vi "SwitchToAnalogOrDigital.vi"(0 "System no.":i32=1 min=1 step=1, 1 "Controller analog board":enum16{"E-711.iA4"}(ring), 2 "Axes to command":string[](array[string]), 3 "Mode":bool=TRUE caption="Mode (Analog:T)", 5 "error in":errorcluster, 6 "AI channels":dbl[](array[numeric]), 7 "AO channels":dbl[](array[numeric]), 8 "Lower voltage limit (V)":dbl=-10.0 format="%.6f", 9 "Upper voltage limit (V)":dbl=10.0 format="%.6f") -> (14 "Conversion factor":dbl[](array[numeric]) format="%.2f", 15 "Offset":dbl[](array[numeric]) format="%#.6f", 19 "Error out":errorcluster)   [LabVIEW 2026]
doc: "This VI sets communication parameters for analog or digital control. Run PI_GCS2_Configuration_Setup.vi prior to running this VI. \n\n- Set System no. to the same value as selected in PI_GCS2_Configuration_Setup.vi. \n- Select the name of the controller analog board (E-711.iA4).\n- Mode can be Analog (T) or Digital (F). \n- Lower voltage limit (V) and Upper voltage limit (V) must match the corresponding settings in Analog_Configuration_Setup.vi, representing the voltage range of the analog input of the controller. The VI checks if the selected values fit into the analog input voltage range of the controller. \n- Axes to command must be a sub set of the axes connected to the controller. \n- AI channels are the analog input channels of the controller to use for analog control. In contrast to the firmware internal names of the analog input channels, select \"1\" here for the first analog input, \"2\" for the second and so on. The VI will automatically determine which input channel names correspond to the selected analog input channels. \n- Similarly, select \"1\" for the first analog output channel (AO channels), \"2\" for the second analog output channel and so on, as the VI will automatically determine which output channel names correspond to the selected analog output channels. \n\nIf the current command level is 0 (CCL?), the VI switches to command level 1 (CCL) before making any further settings and back to 0 afterwards. \nWhen Analog is selected as Mode, the VI connects the selected analog input channels to the selected axes (SPA), sets gain and offset for the analog input (SPA), sets the output type to sensor monitor output (SPA), connects the selected analog output channels to the selected axes (SPA), and sets the position report scaling value and offset for the analog output (SPA).\nWhen Digital is selected as Mode, the VI disconnects the selected analog input channels from the axes (SPA) and sets the output type to control output (SPA).\nThe VI returns the total number of input and output channels available for this controller, the number of sensor input/output channels and the resulting number of analog input/output channels available for analog control. Also, it returns the Gain, Offset and Conversion factor settings resulting from the motion range (TMX?, TMN?) of the selected axes and sets the corresponding parameters (SPA). Finally, it returns the minimum and maximum analog input voltages of the controller as the given lower and upper voltage limits must fit into this range.\n\nSee XXXX_Sample_Application_With_Analog.vi as a sample VI showing how to use this VI in combination with the corresponding Configuration_Setup VIs."
panel:
  out "Max. controller\nanalog input voltage":dbl format="%#.6f"
  out "Min. controller\nanalog input voltage":dbl format="%#.6f"
  out "Gain":dbl[](array[numeric]) format="%#.6f"
  out "No. of output channels":dbl format="%#.0f"
  out "No. of sensor output channels":dbl format="%#.0f"
  out "No. of AO channels":dbl format="%#.0f"
  out "No. of AI channels":dbl format="%#.0f"
  out "No. of sensor input channels":dbl format="%#.0f"
  out "No. of input channels":dbl format="%#.0f"
  # "This VI sets communication parameters for analog or digital control. Run XXXX_Configuration_Setup.vi (with XXXX being the product number of your PI controller) prior to running this VI. Set System no. to the same value as selected in XXXX_Configuration_Setup.vi. See online help for details."
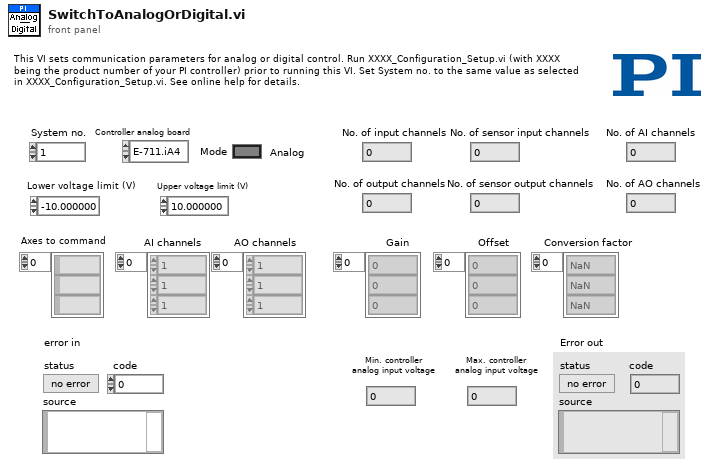
[diagram p1: front panel]
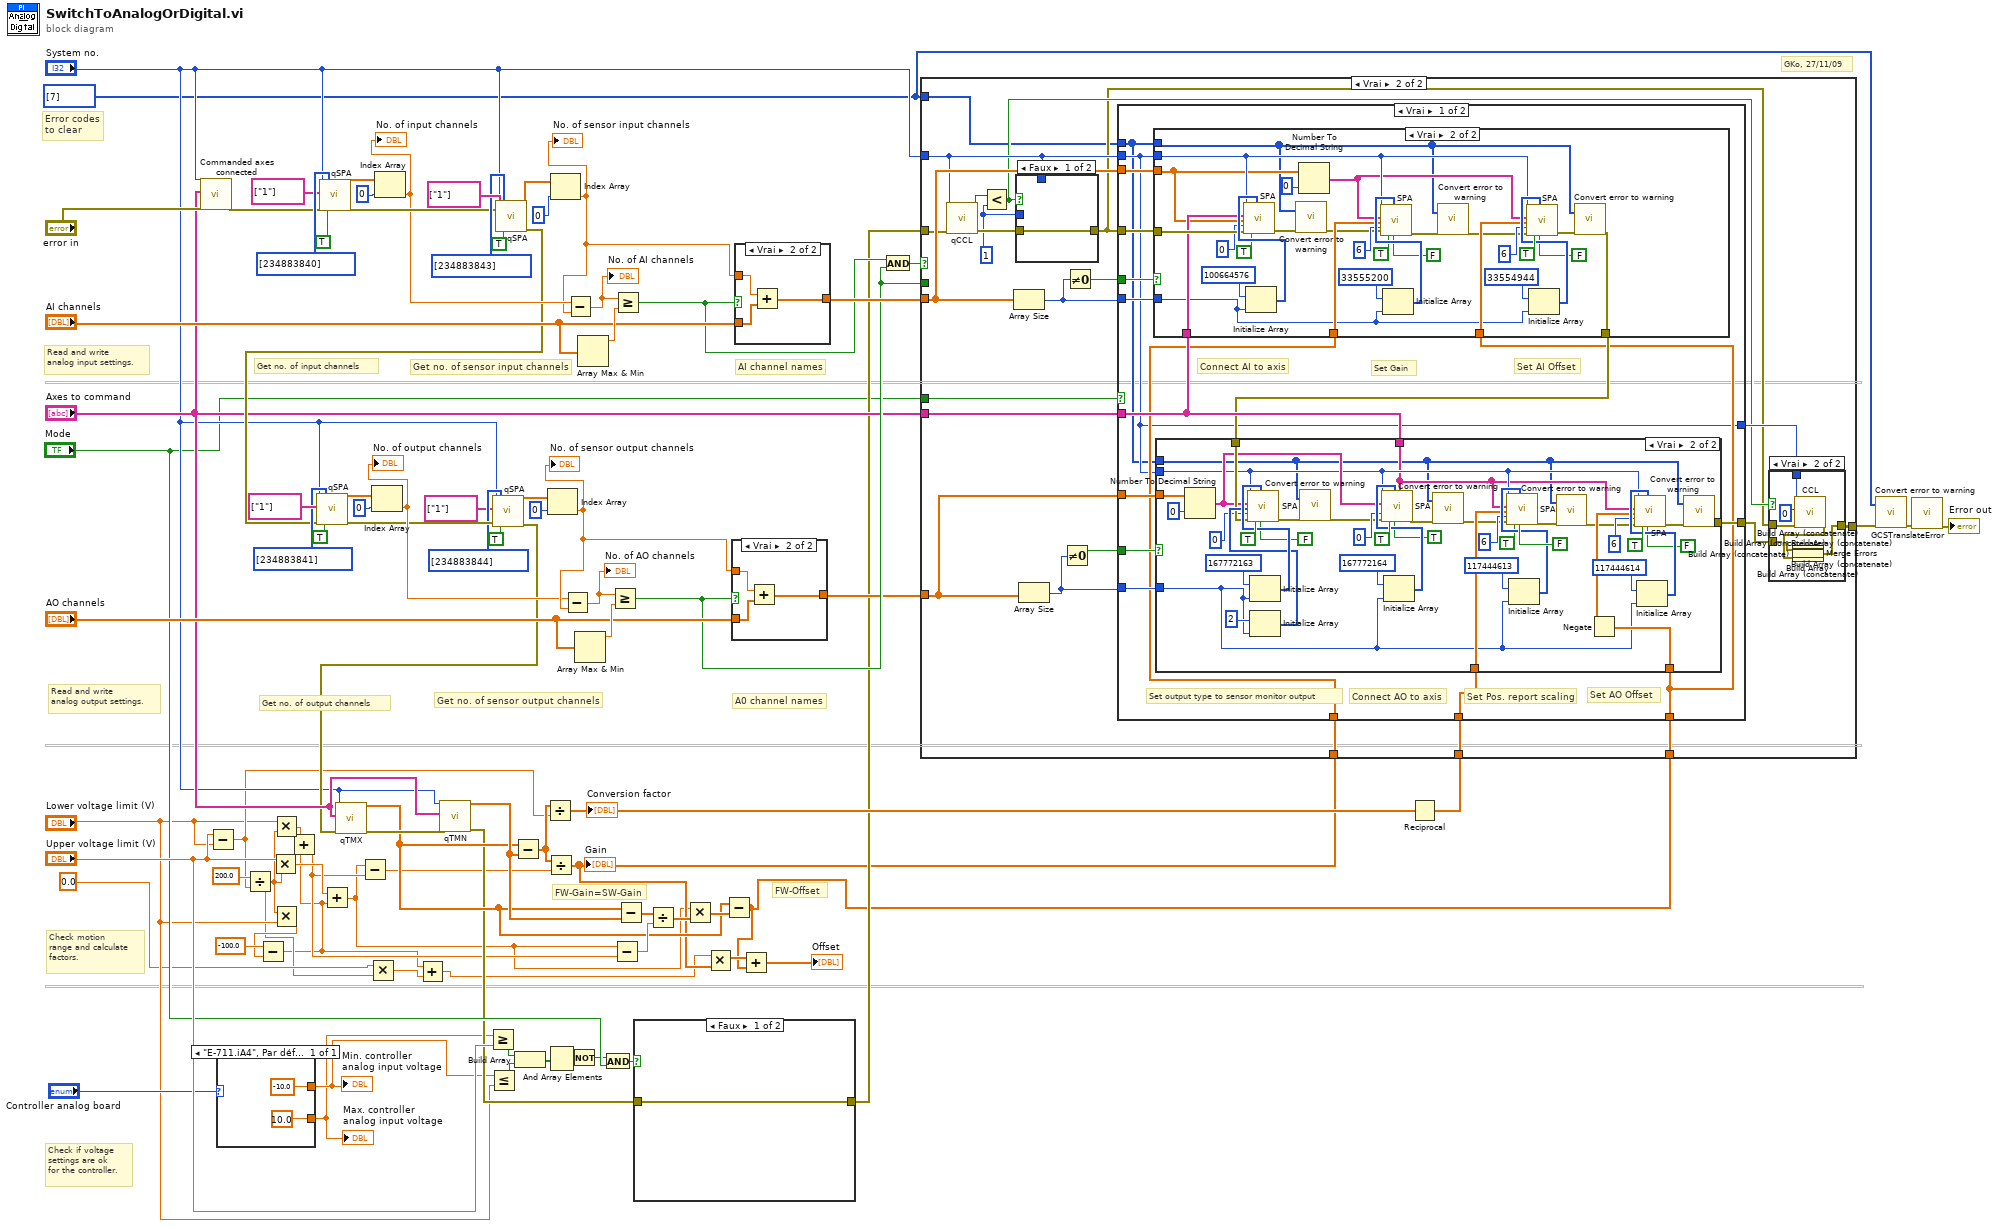
[diagram p0: block diagram]
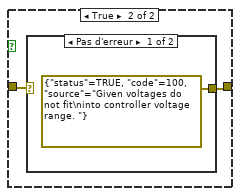
[diagram p2: hidden frame]
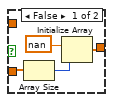
[diagram p4: hidden frame]
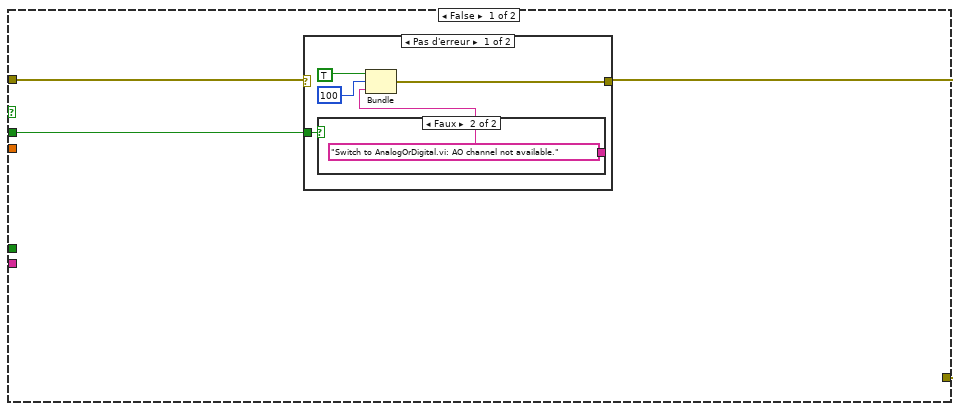
[diagram p5: hidden frame]
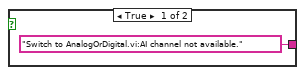
[diagram p6: hidden frame]
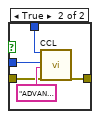
[diagram p9: hidden frame]
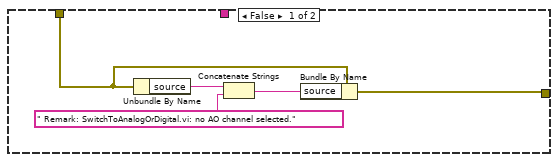
[diagram p10: hidden frame]
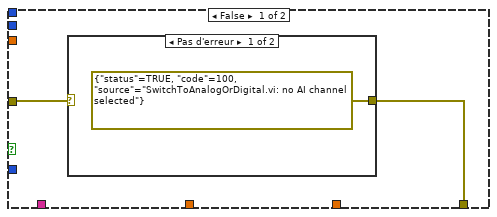
[diagram p11: hidden frame]
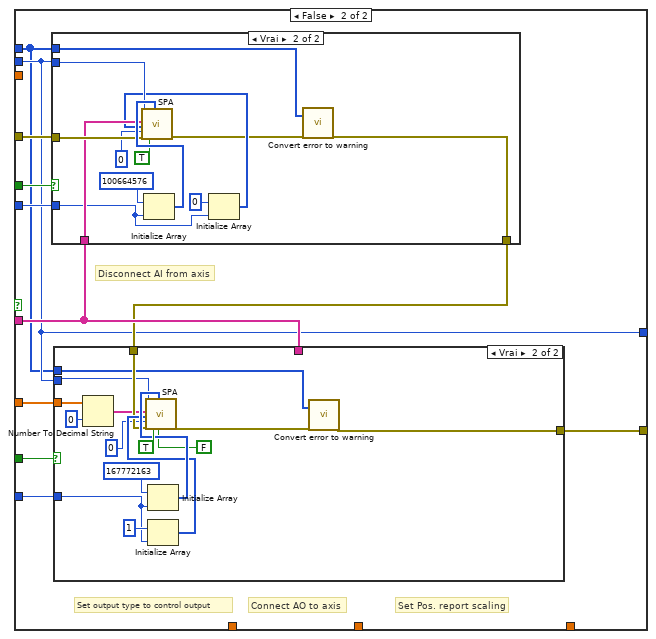
[diagram p13: hidden frame]
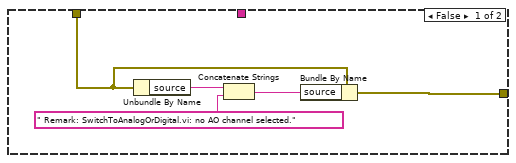
[diagram p14: hidden frame]
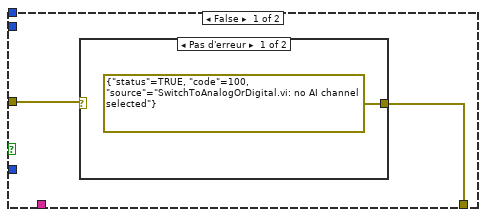
[diagram p15: hidden frame]
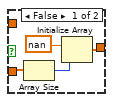
[diagram p17: hidden frame]
diagram:
  w20 = i32[] [7] ("Codes")
  # "Error codes\nto clear"
  # "Get no. of sensor output channels"
  # "Get no. of output channels"
  # "Get no. of sensor input channels"
  # "Get no. of input channels"
  # "FW-Offset"
  # "FW-Gain=SW-Gain"
  # "A0 channel names"
  # "GKo, 27/11/09"
  # "Read and write\nanalog output settings."
  # "Check motion\nrange and calculate\nfactors."
  # "Check if voltage\nsettings are ok\nfor the controller."
  # "AI channel names"
  # "Read and write\nanalog input settings."
  n1 = call "Commanded axes connected.vi"("System no."="System no.", "Commanded axes"="Axes to command", "error in"="error in") -> ("error out"=w73:errorcluster)  [unwired: 16 out]
  n2 = Subtract(x="Upper voltage limit (V)", y="Lower voltage limit (V)") -> (x-y=w18:dbl)
  n3 = case shown="\"E-711.iA4\", Par défaut" "Controller analog board" {
    tunnel: [-10.0 ("y")] -> w25
    tunnel: [10.0 ("y")] -> w24
    frame "E-711.iA4", Default {
    }
  }
  "Min. controller\nanalog input voltage" <- w25
  "Max. controller\nanalog input voltage" <- w24
  n4 = Divide(x=200.0, y=w18) -> (x/y=w3:dbl)
  n5 = Multiply(x="Upper voltage limit (V)", y=w3) -> (x*y=w13:dbl)
  n6 = Multiply(x="Lower voltage limit (V)", y=w3) -> (x*y=w14:dbl)
  n7 = Multiply(x=w3, y="Lower voltage limit (V)") -> (x*y=w15:dbl)
  n8 = Subtract(x=-100.0, y=w15) -> (x-y=w2:dbl)
  n9 = Add(x=w14, y=w2) -> (x+y=w7:dbl)
  n10 = call "qSPA.vi"("System no."="System no.", "Axes to query"=string[] ["1"], "error in"=w73, "Parameter no. (hex)"=u32[] [234883840], "Parameter no. format \n(Decimal: FALSE)"=TRUE ("Parameter no. format \n(Decimal: FALSE)")) -> ("Parameter value"=w86:dbl[], "error out"=w79:errorcluster)  [unwired: 2 in, 11 out]
  n11 = Add(x=w13, y=w2) -> (x+y=w6:dbl)
  n12 = Subtract(x=w6, y=w7) -> (x-y=w4:dbl)
  n13 = Multiply(x=0.0, y=w3) -> (x*y=w5:dbl)
  n14 = Index Array(array=w86, index=0) -> (element=w78:dbl)
  "No. of input channels" <- w78
  n15 = Add(x=w2, y=w5) -> (x+y=w1:dbl)
  n16 = Greater Or Equal?(x=w24, y="Upper voltage limit (V)") -> (x >= y?=w35:bool)
  n17 = Less Or Equal?(x=w25, y="Lower voltage limit (V)") -> (x <= y?=w34:bool)
  n18 = call "qSPA.vi"("System no."="System no.", "Axes to query"=string[] ["1"], "error in"=w79, "Parameter no. (hex)"=u32[] [234883843], "Parameter no. format \n(Decimal: FALSE)"=TRUE ("Parameter no. format \n(Decimal: FALSE)")) -> ("Parameter value"=w83:dbl[], "error out"=w55:errorcluster)  [unwired: 2 in, 11 out]
  n19 = call "qSPA.vi"("System no."="System no.", "Axes to query"=string[] ["1"], "error in"=w55, "Parameter no. (hex)"=u32[] [234883841], "Parameter no. format \n(Decimal: FALSE)"=TRUE ("Parameter no. format \n(Decimal: FALSE)")) -> ("Parameter value"=w59:dbl[], "error out"=w66:errorcluster)  [unwired: 2 in, 11 out]
  n20 = Index Array(array=w59, index=0) -> (element=w67:dbl)
  "No. of output channels" <- w67
  n21 = call "qSPA.vi"("System no."="System no.", "Axes to query"=string[] ["1"], "error in"=w66, "Parameter no. (hex)"=u32[] [234883844], "Parameter no. format \n(Decimal: FALSE)"=TRUE ("Parameter no. format \n(Decimal: FALSE)")) -> ("Parameter value"=w62:dbl[], "error out"=w49:errorcluster)  [unwired: 2 in, 11 out]
  n22 = call "qTMX.vi"("System no."="System no.", "Axes to query"="Axes to command", "error in"=w49) -> ("Maximum travel limit"=w42:dbl[], "error out"=w48:errorcluster)  [unwired: 2 in, 13 out]
  n23 = call "qTMN.vi"("System no."="System no.", "Axes to query"="Axes to command", "error in"=w48) -> ("Minimum travel limit"=w47:dbl[], "error out"=w26:errorcluster)  [unwired: 2 in, 13 out]
  n24 = Subtract(x=w42, y=w47) -> (x-y=w41:dbl[])
  n25 = Build Array(w35, w34) -> (w33:bool[])
  n26 = Divide(x=w41, y=w18) -> (x/y=w40:dbl[])
  "Conversion factor" <- w40
  n27 = Divide(x=w41, y=w4) -> (x/y=w12:dbl[])
  "Gain" <- w12
  n28 = And Array Elements(Boolean array=w33) -> (logical AND=w30:bool)
  n29 = Index Array(array=w62, index=0) -> (element=w68:dbl)
  "No. of sensor output channels" <- w68
  n30 = Index Array(array=w83, index=0) -> (element=w77:dbl)
  "No. of sensor input channels" <- w77
  n31 = Subtract(x=w67, y=w68) -> (x-y=w69:dbl)
  "No. of AO channels" <- w69
  n32 = Subtract(x=w78, y=w77) -> (x-y=w76:dbl)
  "No. of AI channels" <- w76
  n33 = Not(x=w30) -> (.not. x?=w28:bool)
  n34 = Array Max & Min(array="AO channels") -> (max value=w70:dbl)  [unwired: 3 out]
  n35 = Array Max & Min(array="AI channels") -> (max value=w75:dbl)  [unwired: 3 out]
  n36 = And(x=w28, y="Mode") -> (x .and. y?=w27:bool)
  n37 = Greater Or Equal?(x=w69, y=w70) -> (x >= y?=w51:bool)
  n38 = Subtract(x=w6, y=w7) -> (x-y=w45:dbl)
  n39 = Greater Or Equal?(x=w76, y=w75) -> (x >= y?=w53:bool)
  n40 = Subtract(x=w42, y=w47) -> (x-y=w46:dbl[])
  n41 = case shown="Faux" w27 {
    tunnel: w26 -> [w92 w94]
    tunnel: [w92 w93] -> w32
    frame False {
    }
    frame True {
      n42 = case shown="Pas d'erreur" w94 {
        selector: w94 -> [_ w96]
        tunnel: [errorcluster {"status"=TRUE, "code"=100, "source"="Given voltages do not fit\ninto controller voltage range. "} ("error IO") w96] -> w93
        frame No Error {
        }
        frame Error {
        }
      }
    }
  }
  n43 = Divide(x=w46, y=w45) -> (x/y=w44:dbl[])
  n44 = Multiply(x=w6, y=w44) -> (x*y=w43:dbl[])
  n45 = Multiply(x=w1, y=w12) -> (x*y=w11:dbl[])
  n46 = Subtract(x=w42, y=w43) -> (x-y=w10:dbl[])
  n47 = case shown="Vrai" w51 {
    tunnel: "AO channels" -> [w100 w102]
    tunnel: w68 -> [_ w103]
    tunnel: [w97 w101] -> w38
    frame False {
      n48 = Array Size(array=w100) -> (size(s)=w98:i32)
      n49 = Initialize Array(nan, w98) -> (w97:dbl[])
    }
    frame True {
      n50 = Add(x=w103, y=w102) -> (x+y=w101:dbl[])
    }
  }
  n51 = case shown="Vrai" w53 {
    tunnel: "AI channels" -> [w107 w109]
    tunnel: w77 -> [_ w110]
    tunnel: [w104 w108] -> w71
    frame False {
      n52 = Array Size(array=w107) -> (size(s)=w105:i32)
      n53 = Initialize Array(nan, w105) -> (w104:dbl[])
    }
    frame True {
      n54 = Add(x=w110, y=w109) -> (x+y=w108:dbl[])
    }
  }
  n55 = Add(x=w11, y=w10) -> (x+y=→"Offset":dbl[])
  n56 = And(x=w53, y=w51) -> (x .and. y?=w52:bool)
  n57 = Reciprocal(x=w40) -> (1/x=w39:dbl[])
  n58 = case shown="Vrai" w52 {
    tunnel: "System no." -> [_ w128]
    tunnel: w71 -> [_ w133]
    tunnel: "Axes to command" -> [_ w142]
    tunnel: w32 -> [w113 w129]
    tunnel: w51 -> [w112 _]
    tunnel: w38 -> [_ w143]
    tunnel: w12 -> [_ w136]
    tunnel: w10 -> [_ w135]
    tunnel: [w111 w132] -> w22
    tunnel: w39 -> [_ w141]
    tunnel: "Mode" -> [_ w134]
    tunnel: w20 -> [_ w122]
    frame False {
      n59 = case shown="Pas d'erreur" w113 {
        selector: w113 -> [_ w121]
        tunnel: w112 -> [w116 _]
        tunnel: [w114 w121] -> w111
        frame No Error {
          n60 = case shown="Faux" w116 {
            tunnel: ["Switch to AnalogOrDigital.vi:AI channel not available." ("source") "Switch to AnalogOrDigital.vi: AO channel not available." ("source")] -> w115
            frame True {
            }
            frame False {
            }
          }
          n61 = Bundle("status"=TRUE, "code"=100, "source"=w115) -> (w114:errorcluster)  [unwired: 1 out]
        }
        frame Error {
        }
      }
    }
    frame True {
      w126 = 1 ("Command level")
      n62 = call "qCCL.vi"("System no."=w128, "error in"=w129) -> ("Command level"=w127:i32, "error out"=w130:errorcluster)  [unwired: 16 out]
      n63 = Less?(x=w127, y=w126) -> (x < y?=w125:bool)
      n64 = Array Size(array=w133) -> (size(s)=w139:i32)
      n65 = case shown="Faux" w125 {
        tunnel: [w158 w163] -> w124
        tunnel: w130 -> [w158 w161]
        tunnel: w128 -> [_ w160]
        tunnel: w126 -> [_ w159]
        frame False {
        }
        frame True {
          n66 = call "CCL.vi"("System no."=w160, "Command level"=w159, "Password"="ADVANCED", "error in"=w161) -> ("error out"=w163:errorcluster)  [unwired: 15 out]
        }
      }
      n67 = Array Size(array=w143) -> (size(s)=w138:i32)
      n68 = Not Equal To 0?(x=w138) -> (x != 0?=w137:bool)
      n69 = Not Equal To 0?(x=w139) -> (x != 0?=w140:bool)
      n70 = case shown="Vrai" w134 {
        tunnel: w124 -> [w178 w269]
        tunnel: w143 -> [w177 w268]
        tunnel: [w176 w267] -> w123
        tunnel: w142 -> [w175 w266]
        tunnel: w141 -> [w174 _]
        tunnel: w128 -> [w165 w260]
        tunnel: w133 -> [w172 _]
        tunnel: w140 -> [w171 w264]
        tunnel: w139 -> [w170 w263]
        tunnel: w138 -> [w169 w262]
        tunnel: w137 -> [w168 w261]
        tunnel: w136 -> [w167 _]
        tunnel: w135 -> [w166 _]
        tunnel: [w165 w260] -> w131
        tunnel: w122 -> [w164 w259]
        frame True {
          # "Set AO Offset"
          # "Set Pos. report scaling"
          # "Set AI Offset"
          # "Set Gain"
          # "Connect AO to axis"
          # "Set output type to sensor monitor output"
          # "Connect AI to axis"
          n71 = case shown="Vrai" w171 {
            tunnel: w178 -> [w226 w256]
            tunnel: w167 -> [_ w251]
            tunnel: w166 -> [_ w245]
            tunnel: w175 -> [_ w244]
            tunnel: [w225 w230] -> w173
            tunnel: w165 -> [_ w243]
            tunnel: w170 -> [_ w242]
            tunnel: w172 -> [_ w240]
            tunnel: w164 -> [_ w229]
            frame False {
              n72 = case shown="Pas d'erreur" w226 {
                selector: w226 -> [_ w228]
                tunnel: [errorcluster {"status"=TRUE, "code"=100, "source"="SwitchToAnalogOrDigital.vi: no AI channel selected"} ("error IO") w228] -> w225
                frame No Error {
                }
                frame Error {
                }
              }
            }
            frame True {
              n73 = Initialize Array(100664576 ("Numeric"), w242) -> (w257:i32[])
              n74 = call "SPA.vi"("System no."=w243, "Axis to set"=w244, "Parameter value"=w240, "No.of digits"=i16 0, "error in"=w256, "Parameter no. format \n(Decimal: FALSE)"=TRUE ("Parameter no. format \n(Decimal: FALSE)"), "Parameter number (hex)"=w257) -> ("error out"=w235:errorcluster)  [unwired: 3 in, 9 out]
              n75 = call "Convert error to warning.vi"("Codes"=w229, "error in"=w235) -> ("error out"=w234:errorcluster)  [unwired: 17 out]
              n76 = Number To Decimal String(number=w240, width (-)=i16 0) -> (decimal integer string=w241:string[])
              n77 = Initialize Array(33555200 ("Numeric"), w242) -> (w253:i32[])
              n78 = call "SPA.vi"("System no."=w243, "Axis to set"=w241, "Parameter value"=w251, "No.of digits"=i16 6, "error in"=w234, "Parameter no. format \n(Decimal: FALSE)"=TRUE ("Parameter no. format \n(Decimal: FALSE)"), "Parameter number (hex)"=w253, "Parameter format \n(Num.: FALSE)"=FALSE ("Parameter format \n(Num.: FALSE)")) -> ("error out"=w233:errorcluster)  [unwired: 2 in, 9 out]
              n79 = call "Convert error to warning.vi"("Codes"=w229, "error in"=w233) -> ("error out"=w232:errorcluster)  [unwired: 17 out]
              n80 = Initialize Array(33554944 ("Numeric"), w242) -> (w249:i32[])
              n81 = call "SPA.vi"("System no."=w243, "Axis to set"=w241, "Parameter value"=w245, "No.of digits"=i16 6, "error in"=w232, "Parameter no. format \n(Decimal: FALSE)"=TRUE ("Parameter no. format \n(Decimal: FALSE)"), "Parameter number (hex)"=w249, "Parameter format \n(Num.: FALSE)"=FALSE ("Parameter format \n(Num.: FALSE)")) -> ("error out"=w231:errorcluster)  [unwired: 2 in, 9 out]
              n82 = call "Convert error to warning.vi"("Codes"=w229, "error in"=w231) -> ("error out"=w230:errorcluster)  [unwired: 17 out]
            }
          }
          n83 = case shown="Vrai" w168 {
            tunnel: w177 -> [_ w216]
            tunnel: [w179 w185] -> w176
            tunnel: w175 -> [_ w198]
            tunnel: w174 -> [_ w209]
            tunnel: w173 -> [w180 w208]
            tunnel: w165 -> [_ w201]
            tunnel: w169 -> [_ w193]
            tunnel: w166 -> [_ w200]
            tunnel: w164 -> [_ w184]
            frame False {
              n84 = Unbundle By Name(w180) -> ("source"=w183:string)
              n85 = Concatenate Strings(w183, " Remark: SwitchToAnalogOrDigital.vi: no AO channel selected." ("source")) -> (w181:string)
              n86 = Bundle By Name(cluster=w180, "source"=w181) -> (w179:errorcluster)
            }
            frame True {
              n87 = Number To Decimal String(number=w216, width (-)=i16 0) -> (decimal integer string=w207:string[])
              n88 = Initialize Array(167772163 ("Numeric"), w193) -> (w223:i32[])
              n89 = Initialize Array(2 ("element"), w193) -> (w220:i32[])
              n90 = call "SPA.vi"("System no."=w201, "Axis to set"=w207, "Parameter value"=w220, "No.of digits"=i16 0, "error in"=w208, "Parameter no. format \n(Decimal: FALSE)"=TRUE ("Parameter no. format \n(Decimal: FALSE)"), "Parameter number (hex)"=w223, "Parameter format \n(Num.: FALSE)"=FALSE ("Parameter format \n(Num.: FALSE)")) -> ("error out"=w192:errorcluster)  [unwired: 2 in, 9 out]
              n91 = call "Convert error to warning.vi"("Codes"=w184, "error in"=w192) -> ("error out"=w191:errorcluster)  [unwired: 17 out]
              n92 = Initialize Array(167772164 ("Numeric"), w193) -> (w218:i32[])
              n93 = call "SPA.vi"("System no."=w201, "Axis to set"=w207, "No.of digits"=i16 0, "error in"=w191, "Parameter no. format \n(Decimal: FALSE)"=TRUE ("Parameter no. format \n(Decimal: FALSE)"), "Parameter number (hex)"=w218, "Parameter format \n(Num.: FALSE)"=TRUE ("Parameter format \n(Num.: FALSE)"), "Parameter string"=w198) -> ("error out"=w190:errorcluster)  [unwired: 2 in, 9 out]
              n94 = call "Convert error to warning.vi"("Codes"=w184, "error in"=w190) -> ("error out"=w189:errorcluster)  [unwired: 17 out]
              n95 = Initialize Array(117444613 ("Numeric"), w193) -> (w211:i32[])
              n96 = call "SPA.vi"("System no."=w201, "Axis to set"=w198, "Parameter value"=w209, "No.of digits"=i16 6, "error in"=w189, "Parameter no. format \n(Decimal: FALSE)"=TRUE ("Parameter no. format \n(Decimal: FALSE)"), "Parameter number (hex)"=w211, "Parameter format \n(Num.: FALSE)"=FALSE ("Parameter format \n(Num.: FALSE)")) -> ("error out"=w187:errorcluster)  [unwired: 2 in, 9 out]
              n97 = call "Convert error to warning.vi"("Codes"=w184, "error in"=w187) -> ("error out"=w188:errorcluster)  [unwired: 17 out]
              n98 = Negate(x=w200) -> (-x=w199:dbl[])
              n99 = Initialize Array(117444614 ("Numeric"), w193) -> (w204:i32[])
              n100 = call "SPA.vi"("System no."=w201, "Axis to set"=w198, "Parameter value"=w199, "No.of digits"=i16 6, "error in"=w188, "Parameter no. format \n(Decimal: FALSE)"=TRUE ("Parameter no. format \n(Decimal: FALSE)"), "Parameter number (hex)"=w204, "Parameter format \n(Num.: FALSE)"=FALSE ("Parameter format \n(Num.: FALSE)")) -> ("error out"=w186:errorcluster)  [unwired: 2 in, 9 out]
              n101 = call "Convert error to warning.vi"("Codes"=w184, "error in"=w186) -> ("error out"=w185:errorcluster)  [unwired: 17 out]
            }
          }
        }
        frame False {
          # "Set Pos. report scaling"
          # "Connect AO to axis"
          # "Set output type to control output"
          # "Disconnect AI from axis"
          n102 = case shown="Vrai" w264 {
            tunnel: w269 -> [w292 w305]
            tunnel: w266 -> [_ w303]
            tunnel: [w291 w297] -> w265
            tunnel: w260 -> [_ w302]
            tunnel: w263 -> [_ w301]
            tunnel: w259 -> [_ w295]
            frame False {
              n103 = case shown="Pas d'erreur" w292 {
                selector: w292 -> [_ w294]
                tunnel: [errorcluster {"status"=TRUE, "code"=100, "source"="SwitchToAnalogOrDigital.vi: no AI channel selected"} ("error IO") w294] -> w291
                frame No Error {
                }
                frame Error {
                }
              }
            }
            frame True {
              n104 = Initialize Array(100664576 ("Numeric"), w301) -> (w306:i32[])
              n105 = Initialize Array(0 ("element"), w301) -> (w299:i32[])
              n106 = call "SPA.vi"("System no."=w302, "Axis to set"=w303, "Parameter value"=w299, "No.of digits"=i16 0, "error in"=w305, "Parameter no. format \n(Decimal: FALSE)"=TRUE ("Parameter no. format \n(Decimal: FALSE)"), "Parameter number (hex)"=w306) -> ("error out"=w296:errorcluster)  [unwired: 3 in, 9 out]
              n107 = call "Convert error to warning.vi"("Codes"=w295, "error in"=w296) -> ("error out"=w297:errorcluster)  [unwired: 17 out]
            }
          }
          n108 = case shown="Vrai" w261 {
            tunnel: w268 -> [_ w285]
            tunnel: [w270 w277] -> w267
            tunnel: w266 -> [_ _]
            tunnel: w265 -> [w274 w283]
            tunnel: w260 -> [_ w282]
            tunnel: w262 -> [_ w281]
            tunnel: w259 -> [_ w275]
            frame False {
              n109 = Unbundle By Name(w274) -> ("source"=w273:string)
              n110 = Concatenate Strings(w273, " Remark: SwitchToAnalogOrDigital.vi: no AO channel selected." ("source")) -> (w271:string)
              n111 = Bundle By Name(cluster=w274, "source"=w271) -> (w270:errorcluster)
            }
            frame True {
              n112 = Number To Decimal String(number=w285, width (-)=i16 0) -> (decimal integer string=w280:string[])
              n113 = Initialize Array(167772163 ("Numeric"), w281) -> (w289:i32[])
              n114 = Initialize Array(1 ("element"), w281) -> (w286:i32[])
              n115 = call "SPA.vi"("System no."=w282, "Axis to set"=w280, "Parameter value"=w286, "No.of digits"=i16 0, "error in"=w283, "Parameter no. format \n(Decimal: FALSE)"=TRUE ("Parameter no. format \n(Decimal: FALSE)"), "Parameter number (hex)"=w289, "Parameter format \n(Num.: FALSE)"=FALSE ("Parameter format \n(Num.: FALSE)")) -> ("error out"=w276:errorcluster)  [unwired: 2 in, 9 out]
              n116 = call "Convert error to warning.vi"("Codes"=w275, "error in"=w276) -> ("error out"=w277:errorcluster)  [unwired: 17 out]
            }
          }
        }
      }
      n117 = case shown="Vrai" w125 {
        tunnel: [w144 w152] -> w132
        tunnel: w131 -> [_ w157]
        tunnel: w124 -> [_ w155]
        tunnel: w123 -> [w144 w153]
        frame False {
        }
        frame True {
          n118 = call "CCL.vi"("System no."=w157, "Command level"=0, "error in"=w155) -> ("error out"=w154:errorcluster)  [unwired: 1 in, 15 out]
          n119 = Build Array(w153, w154) -> (w151:errorcluster[])
          n120 = Build Array (concatenate)(w151) -> (w150:errorcluster[])
          n121 = Build Array (concatenate)(w150) -> (w149:errorcluster[])
          n122 = Build Array (concatenate)(w149) -> (w148:errorcluster[])
          n123 = Build Array (concatenate)(w148) -> (w147:errorcluster[])
          n124 = Build Array (concatenate)(w147) -> (w146:errorcluster[])
          n125 = Build Array (concatenate)(w146) -> (w145:errorcluster[])
          n126 = Merge Errors(w145) -> (w152:errorcluster)
        }
      }
    }
  }
  n127 = call "Convert error to warning.vi"("Codes"=w20, "error in"=w22) -> ("error out"=w21:errorcluster)  [unwired: 17 out]
  n128 = call "GCSTranslateError.vi"("error in"=w21) -> ("error out"=→"Error out":errorcluster)  [unwired: 18 out]
